vi "ResetFlowMeter.vi"(5 "Initialize?":bool, 7 "FVIR?":bool, 8 "error in (no error)":errorcluster, 11 "Modbus Queue in":refnum<queue>) -> (0 "error out":errorcluster, 3 "dup Message Queue":refnum<queue>)   [LabVIEW 2023]
uses:
  Message Queue/Message Cluster.ctl
  Message Queue/Enqueue Message (Single).vi
  Message Queue/Message Queue.lvlib
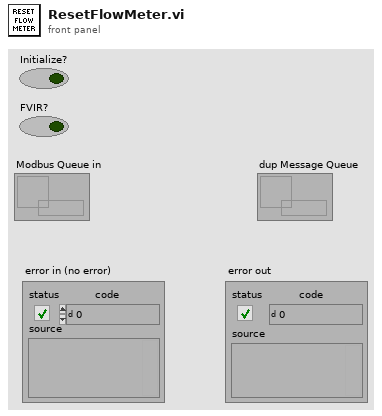
[diagram p1: front panel]
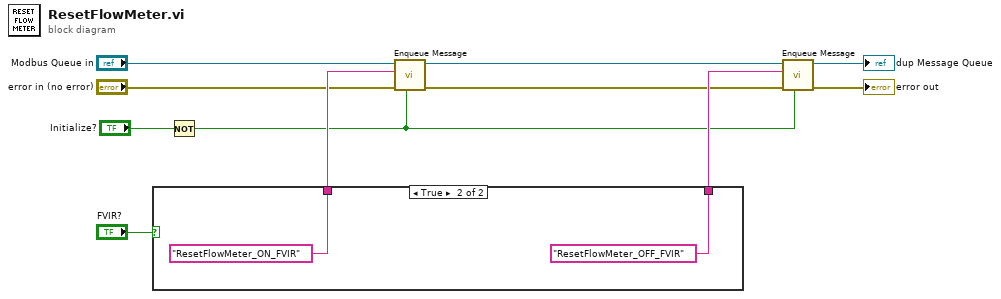
[diagram p0: block diagram]
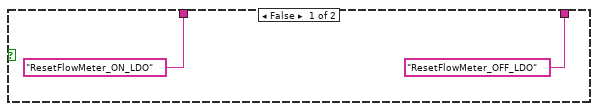
[diagram p2: hidden frame]
diagram:
  n1 = case shown="True" "FVIR?" {
    tunnel: ["ResetFlowMeter_ON_LDO" ("Message") "ResetFlowMeter_ON_FVIR" ("Message")] -> w10
    tunnel: ["ResetFlowMeter_OFF_LDO" ("Message") "ResetFlowMeter_OFF_FVIR" ("Message")] -> w9
    frame False {
    }
    frame True {
    }
  }
  n2 = Not(x="Initialize?") -> (.not. x?=w3:bool)
  n3 = call-poly "Enqueue Message.vi"("Priority Message? (F)"=w3, "error in (no error)"="error in (no error)", "Message"=w10, "Message Queue"="Modbus Queue in") -> ("error out"=w1:errorcluster, "dup Message Queue"=w8:refnum<queue>)  [unwired: 6 in]
  n4 = call-poly "Enqueue Message.vi"("Priority Message? (F)"=w3, "error in (no error)"=w1, "Message"=w9, "Message Queue"=w8) -> ("error out"=→"error out":errorcluster, "dup Message Queue"=→"dup Message Queue":refnum<queue>)  [unwired: 6 in]
